vi "Write Timeout.vi"(8 "error in (no error)":errorcluster, 10 "Timeout":i32=10000, 11 "REST Client_NET in":refnum<class "REST Client_NET.lvclass">) -> (0 "error out":errorcluster, 3 "REST Client_NET out":refnum<class "REST Client_NET.lvclass">)   [LabVIEW 2018, in "REST Client_NET.lvlib" / "REST Client_NET.lvclass"]
doc: "Write Timeout value\n<b> </b> <b> </b>\nHttpClient_NET\nJustin Young - Viviota\nCopyright (c) 2021\nLicense: BSD"
uses:
  REST Client_NET.lvclass
  REST Client_NET.lvclass/REST Client_NET.ctl
  classes/REST Client/REST Client.lvclass
  LabVIEWHTTPClient_NET/HttpClient_NET.lvclass
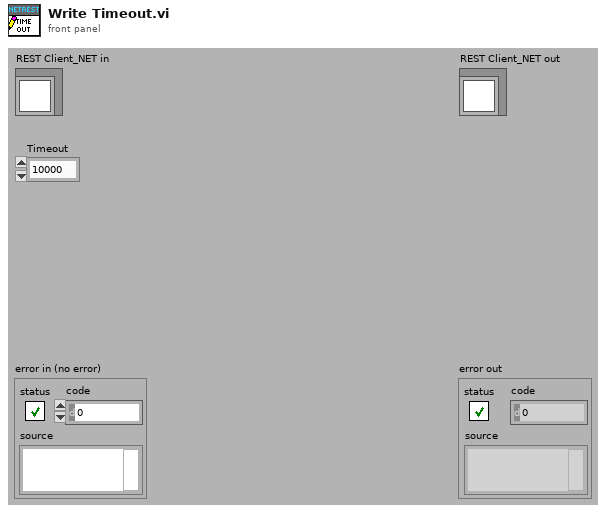
[diagram p1: front panel]
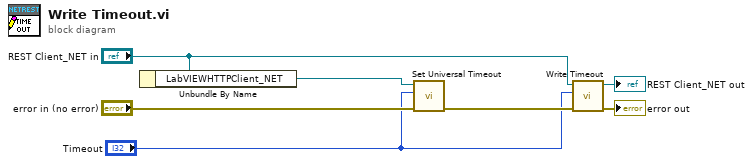
[diagram p0: block diagram]
diagram:
  n1 = Unbundle By Name("REST Client_NET in") -> ("LabVIEWHTTPClient_NET"=w4:refnum<class "HttpClient_NET.lvclass">)
  n2 = call "Set Universal Timeout.vi"("error in (no error)"="error in (no error)", "timeout_ms (10000)"="Timeout", "LabVIEWHTTPClient_NET in"=w4) -> ("error out"=w2:errorcluster)  [unwired: 7 in, 1 out]
  n3 = call-parent "Write Timeout.vi"("error in (no error)"=w2, "Timeout"="Timeout", "REST Client in"="REST Client_NET in") -> ("error out"=→"error out":errorcluster, "REST Client out"=→"REST Client_NET out":refnum<class "REST Client_NET.lvclass">)  [unwired: 7 in]
